vi "CIMAQ_GetHighlightKernel.vi"(11 "n":u8=7) -> (3 "Highlight Kernel":sgl[][](array[numeric]))   [LabVIEW 2017]
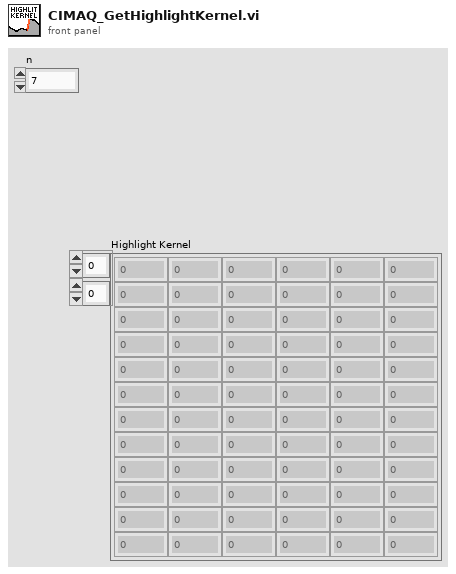
[diagram p1: front panel]
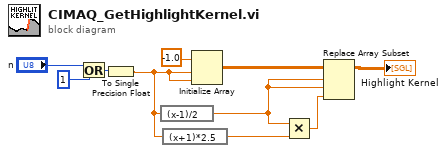
[diagram p0: block diagram]
diagram:
  n1 = Or(x="n", y=u8 1) -> (x .or. y?=w2:u8)
  n2 = To Single Precision Float(number=w2) -> (single precision float=w1:sgl)
  n3 = expression code="(x-1)/2"(w1) -> (w6:sgl)
  n4 = expression code="(x+1)*2.5"(w1) -> (w5:sgl)
  n5 = Initialize Array "Initialize Array"(sgl -1.0, w1, w1) -> (w7:sgl[][])
  n6 = Multiply(x=w6, y=w5) -> (x*y=w4:sgl)
  n7 = Replace Array Subset(array=w7, new element=w4, index (row)=w6, index (col)=w6) -> (→"Highlight Kernel":sgl[][])
